vi "Process Template Graphics.vi"(8 "error in (no error)":errorcluster, 10 "Data":cluster{T1[], i32, bool}, 11 "Data in":T2={"Class"={"Ants"=refnum, "Layer"=refnum, "Templates"=refnum, "Icon"=refnum, "Glyph"=refnum, "Settings"=refnum, "Tools"=refnum}, "Ref"={"Add Layer"=refnum, "Remove Layer"=refnum, "Line Text"=[], "Body Text Spec"=refnum, "DNL_Font"=refnum, "glyph path str"=refnum, "templates path str"=refnum, "Arrow Up"=refnum, "Arrow Down"=refnum, "IE VI Ref"=refnum, "Glyphs tree"=refnum, "Templates tree"=refnum, "Layer Icon Text"=refnum, "Layer Template"=refnum, "Clipboard"=refnum, "BW icon in"=refnum, "Color icon in"=refnum, "Layer Clust"=refnum, "Body Text"=refnum, "DNL_Framework Templates"=refnum, "Search Templates"=refnum, "TextMarker"=refnum, "Tab Control"=refnum, "Search Glyphs"=refnum, "Line Color"=refnum, "DNL_Glyphs []"=refnum, "Fill Color"=refnum, "Tools"=refnum, "Glyphs tree"=refnum, "Icon"=refnum, "Preview"=refnum, "Ants"=refnum, "Terminals"=refnum, "menu reference"=refnum, "LayerNames"=[], "GlyphLoadAnimation"=refnum, "TemplateLoadAnimation"=refnum, "refreshGlyphs"=refnum, "refreshTemplates"=refnum}, "Support"={"AntsRect"={"left"=0, "top"=0, "right"=0, "bottom"=0}, "Mouse Move Coords"={"Horizontal"=0, "Vertical"=0}, "Mouse Down Coords"={"Horizontal"=0, "Vertical"=0}, "Temp Coord"={"Horizontal"=0, "Vertical"=0}, "Action"=enum."Default", "Edge Color"=4914962, "Fill Color"=16860, "Mouse Down?"=FALSE, "Draft Mode?"=FALSE, "Temp Icon"=bytes[3102], "CTRL Pressed"=FALSE, "Move Selection?"=FALSE, "AntsRect Orig"={"left"=0, "top"=0, "right"=0, "bottom"=0}, "Text"="", "TM Set?"=FALSE, "Mouse inside icon?"=FALSE, "Tool (old value)"=0, "Pencil Move Color"=0, "Swap Colors?"=FALSE, "Shift pressed?"=FALSE}}) -> (0 "error out":errorcluster, 3 "Data out":T2={"Class"={"Ants"=refnum, "Layer"=refnum, "Templates"=refnum, "Icon"=refnum, "Glyph"=refnum, "Settings"=refnum, "Tools"=refnum}, "Ref"={"Add Layer"=refnum, "Remove Layer"=refnum, "Line Text"=[], "Body Text Spec"=refnum, "DNL_Font"=refnum, "glyph path str"=refnum, "templates path str"=refnum, "Arrow Up"=refnum, "Arrow Down"=refnum, "IE VI Ref"=refnum, "Glyphs tree"=refnum, "Templates tree"=refnum, "Layer Icon Text"=refnum, "Layer Template"=refnum, "Clipboard"=refnum, "BW icon in"=refnum, "Color icon in"=refnum, "Layer Clust"=refnum, "Body Text"=refnum, "DNL_Framework Templates"=refnum, "Search Templates"=refnum, "TextMarker"=refnum, "Tab Control"=refnum, "Search Glyphs"=refnum, "Line Color"=refnum, "DNL_Glyphs []"=refnum, "Fill Color"=refnum, "Tools"=refnum, "Glyphs tree"=refnum, "Icon"=refnum, "Preview"=refnum, "Ants"=refnum, "Terminals"=refnum, "menu reference"=refnum, "LayerNames"=[], "GlyphLoadAnimation"=refnum, "TemplateLoadAnimation"=refnum, "refreshGlyphs"=refnum, "refreshTemplates"=refnum}, "Support"={"AntsRect"={"left"=0, "top"=0, "right"=0, "bottom"=0}, "Mouse Move Coords"={"Horizontal"=0, "Vertical"=0}, "Mouse Down Coords"={"Horizontal"=0, "Vertical"=0}, "Temp Coord"={"Horizontal"=0, "Vertical"=0}, "Action"=enum."Default", "Edge Color"=4914962, "Fill Color"=16860, "Mouse Down?"=FALSE, "Draft Mode?"=FALSE, "Temp Icon"=bytes[3102], "CTRL Pressed"=FALSE, "Move Selection?"=FALSE, "AntsRect Orig"={"left"=0, "top"=0, "right"=0, "bottom"=0}, "Text"="", "TM Set?"=FALSE, "Mouse inside icon?"=FALSE, "Tool (old value)"=0, "Pencil Move Color"=0, "Swap Colors?"=FALSE, "Shift pressed?"=FALSE}})   [LabVIEW 2021, in "FakedArray.lvclass"]
uses:
  FakedArray.lvclass
  vi.lib/LabVIEW Icon API/lv_icon/Controls/Graphic.ctl
  Controls/IE Data.ctl
  Ants/Ants.lvclass
  vi.lib/LabVIEW Icon API/lv_icon/Classes/Icon/Icon.lvclass
  Icon Library/Glyph.lvclass
  Settings/Settings.lvclass
  Tools/Tools Paint.lvclass
  Controls/IE Classes.ctl
  Controls/References Cluster.ctl
  Controls/SupportClass.ctl
  <vilib>/Utility/miscctls.llb/LVPoint32TypeDef.ctl
  Controls/SupportClass_Action.ctl
  vi.lib/LabVIEW Icon API/lv_icon/Controls/IEColor.ctl
  Global Variables/Data.vi
panel:
  in  "?":T1
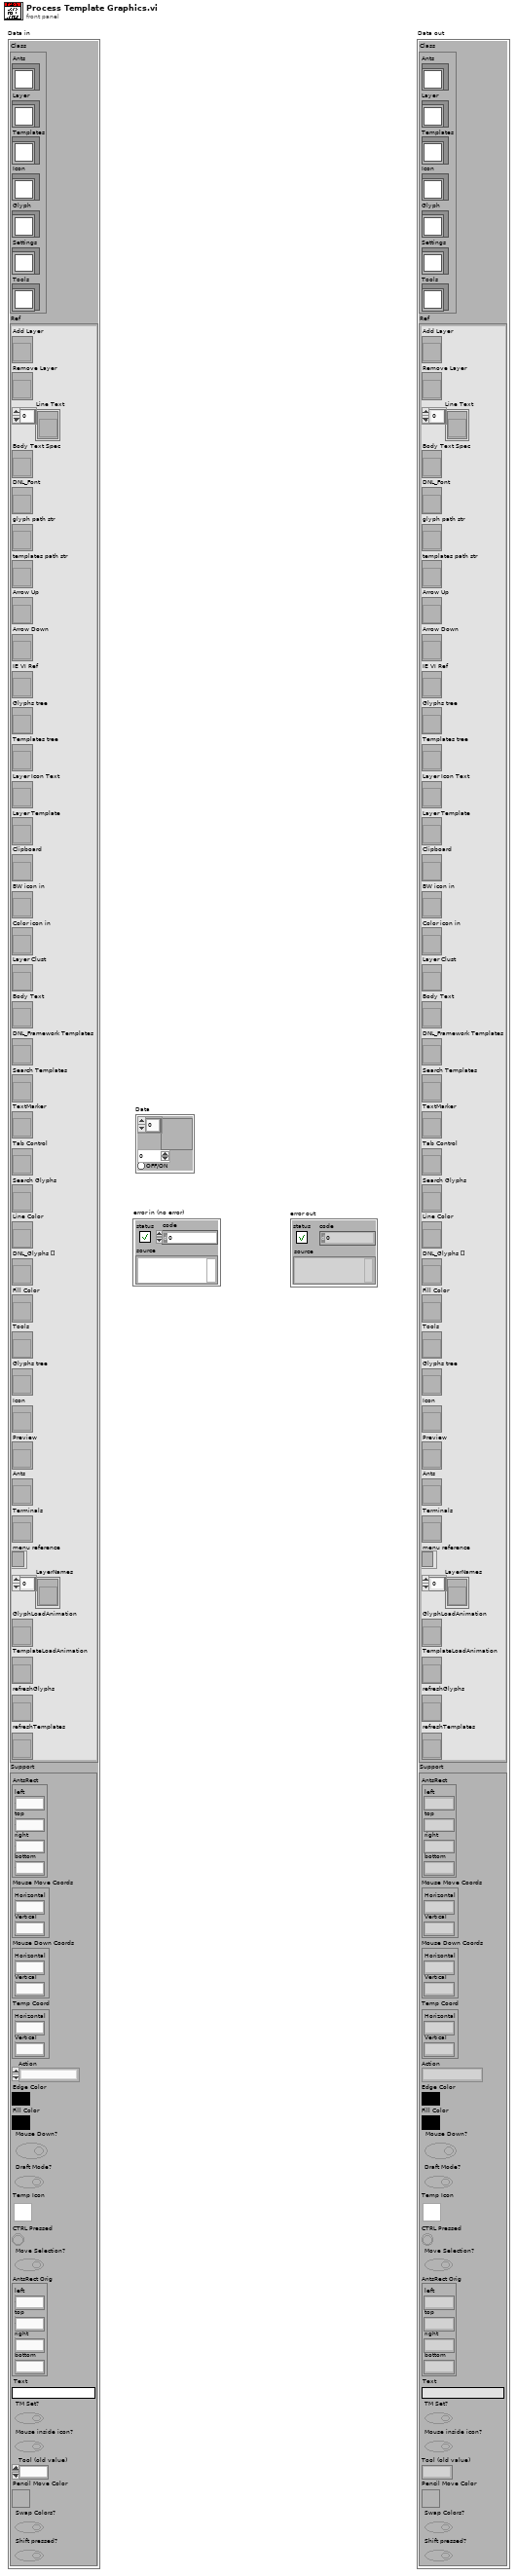
[diagram p1: front panel]
types:
  T1 = typedef "Graphic.ctl" = cluster{"Rectangle":cluster{"left":i16, "top":i16, "right":i16, "bottom":i16}, "Path":path, "Image":picture, "Filter":string, "FileName":string}
  T2 = typedef "IE Data.ctl" = cluster{"Class":T3, "Ref":T4, "Support":T5}
  T3 = typedef "IE Classes.ctl" = cluster{"Ants":refnum<class "Ants.lvclass">, "Layer":refnum<class "FakedArray.lvclass">, "Templates":refnum<class "FakedArray.lvclass">, "Icon":refnum<class "Icon.lvclass">, "Glyph":refnum<class "Glyph.lvclass">, "Settings":refnum<class "Settings.lvclass">, "Tools":refnum<class "Tools Paint.lvclass">}
  T4 = typedef "References Cluster.ctl" = cluster{"Add Layer":refnum<vi>, "Remove Layer":refnum<vi>, "Line Text":refnum<vi>[], "Body Text Spec":refnum<vi>, "DNL_Font":refnum<vi>, "glyph path str":refnum<vi>, "templates path str":refnum<vi>, "Arrow Up":refnum<vi>, "Arrow Down":refnum<vi>, "IE VI Ref":refnum<vi>, "Glyphs tree":refnum<vi>, "Templates tree":refnum<vi>, "Layer Icon Text":refnum<vi>, "Layer Template":refnum<vi>, "Clipboard":refnum<vi>, "BW icon in":refnum<vi>, "Color icon in":refnum<vi>, "Layer Clust":refnum<vi>, "Body Text":refnum<vi>, "DNL_Framework Templates":refnum<vi>, "Search Templates":refnum<vi>, "TextMarker":refnum<vi>, "Tab Control":refnum<vi>, "Search Glyphs":refnum<vi>, "Line Color":refnum<vi>, "DNL_Glyphs []":refnum<vi>, "Fill Color":refnum<vi>, "Tools":refnum<vi>, "Glyphs tree":refnum<vi>, "Icon":refnum<vi>, "Preview":refnum<vi>, "Ants":refnum<vi>, "Terminals":refnum<vi>, "menu reference":refnum<k9>, "LayerNames":refnum<vi>[], "GlyphLoadAnimation":refnum<vi>, "TemplateLoadAnimation":refnum<vi>, "refreshGlyphs":refnum<vi>, "refreshTemplates":refnum<vi>}
  T5 = typedef "SupportClass.ctl" = cluster{"AntsRect":cluster{"left":i16, "top":i16, "right":i16, "bottom":i16}, "Mouse Move Coords":T6, "Mouse Down Coords":T6, "Temp Coord":T6, "Action":T7, "Edge Color":T8, "Fill Color":T8, "Mouse Down?":bool, "Draft Mode?":bool, "Temp Icon":picture, "CTRL Pressed":bool, "Move Selection?":bool, "AntsRect Orig":cluster{"left":i16, "top":i16, "right":i16, "bottom":i16}, "Text":string, "TM Set?":bool, "Mouse inside icon?":bool, "Tool (old value)":u32, "Pencil Move Color":u32, "Swap Colors?":bool, "Shift pressed?":bool}
  T6 = typedef "LVPoint32TypeDef.ctl" = cluster{"Horizontal":i32, "Vertical":i32}
  T7 = typedef "SupportClass_Action.ctl" = enum16{"Default", "Move Selection", "Glyph Library", "Tool"}
  T8 = typedef "IEColor.ctl" = u32
  T9 = typedef "Path&Icon.ctl" = cluster{"Rectangle":cluster{"left":i16, "top":i16, "right":i16, "bottom":i16}, "Path":path, "Image":picture, "Filter":string, "FileName":string}
  T10 = typedef "Icon Editor Invoker Type.ctl" = enum32{"Unknown Icon Source", "VI Icon", "Library Icon (any library type)", "Palette icon", "Icon from App Method"}
  T11 = typedef "Pathes.ctl" = enum16{"Root Path", "Icon Templates", "Icon Templates VI", "Icon Templates Lib", "Glyphs"}
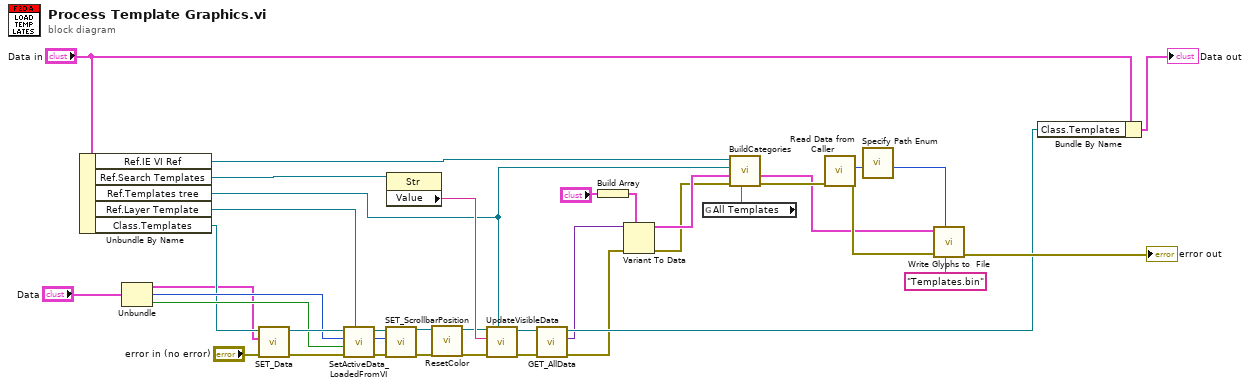
[diagram p0: block diagram]
diagram:
  n1 = Unbundle By Name("Data in") -> ("Ref.IE VI Ref"=w14:refnum<vi>, "Ref.Search Templates"=w22:refnum<vi>, "Ref.Templates tree"=w15:refnum<vi>, "Ref.Layer Template"=w17:refnum<vi>, "Class.Templates"=w21:refnum<class "FakedArray.lvclass">)
  n2 = Unbundle("Data") -> (w16:T1[], w35:i32, w34:bool)
  n3 = call-dynamic "SET_Data.vi"("error in (no error)"="error in (no error)", "Data"=w16, "FakedArray in"=w21) -> ("error out"=w37:errorcluster, "FakedArray out"=w38:refnum<class "FakedArray.lvclass">)  [unwired: 7 out]
  n4 = call "SetActiveData_LoadedFromVI.vi"("Layer Template"=w17, "error in (no error)"=w37, "Match?"=w34, "Match Index"=w35, "FakedArray in"=w38) -> ("error out"=w31:errorcluster, "Position Scrollbar"=w30:i32, "FakedArray out"=w32:refnum<class "FakedArray.lvclass">)  [unwired: 4 out]
  n5 = call-dynamic "SET_ScrollbarPosition.vi"("error in (no error)"=w31, "Scrollbar Position"=w30, "FakedArray.lvclass in"=w32) -> ("error out"=w26:errorcluster, "FakedArray.lvclass out"=w25:refnum<class "FakedArray.lvclass">)  [unwired: 7 out]
  n6 = property class="Str"(reference=w22) -> ("Value"=w27:string)  [unwired: 1 in, 2 out]
  n7 = call "ResetColor.vi"("error in (no error)"=w26, "FakedArray in"=w25) -> ("error out"=w23:errorcluster, "FakedArray out"=w24:refnum<class "FakedArray.lvclass">)  [unwired: 8 out]
  n8 = call-dynamic "UpdateVisibleData.vi"("Templates tree"=w15, "error in (no error)"=w23, "Keyword"=w27, "FakedArray in"=w24) -> ("error out"=w11:errorcluster, "FakedArray out"=w12:refnum<class "FakedArray.lvclass">)  [unwired: 1 in, 5 out]
  n9 = call-dynamic "GET_AllData.vi"("error in (no error)"=w11, "FakedArray.lvclass in"=w12) -> ("error out"=w5:errorcluster, "Data"=w7:variant, "FakedArray.lvclass out"=w10:refnum<class "FakedArray.lvclass">)  [unwired: 7 out]
  n10 = Build Array("?") -> (w8:T1[])
  n11 = Variant To Data(error in=w5, type=w8, Variant=w7) -> (data=w6:T1[], error out=w4:errorcluster)
  n12 = global read "Data.vi" "All Templates"() -> (w29:string)
  n13 = call "BuildCategories.vi"("Main Item"=w29, "error in (no error)"=w4, "IconTemplates in"=w6, "Tree"=w15, "VI IE Ref"=w14) -> ("error out"=w28:errorcluster, "IconTemplates out"=w1:T9[])  [unwired: 5 out]
  n14 = call "Read Data from Caller.vi"("error in (no error)"=w28) -> ("error out"=w13:errorcluster, "Icon Editor Invoker Type"=w3:T10)  [unwired: 2 in, 7 out]
  n15 = call "Specify Path Enum.vi"("Icon Editor Invoker Type"=w3) -> ("Path"=w2:T11)  [unwired: 10 out]
  n16 = call "Write Glyphs to  File.vi"("File Name"="Templates.bin", "Path"=w2, "error in (no error)"=w13, "Graphics []"=w1) -> ("error out"=→"error out":errorcluster)  [unwired: 7 out]
  n17 = Bundle By Name(cluster="Data in", "Class.Templates"=w10) -> (→"Data out":T2)
